vi "ArmPressureCalcMethod.vi"() -> ()   [LabVIEW 2013]
uses:
  Controls/Enum Save Action Events.ctl
  main.lvlib
panel:
  in  "SaveBtn":bool
  out "Description":string="Beregner det gennemsnitlige tryk ud fra alle de indtastede værdier for hver kolonne. "
  in  "Calculation Type":T1(ring) caption="Vælg metode til udregning af amtryk"
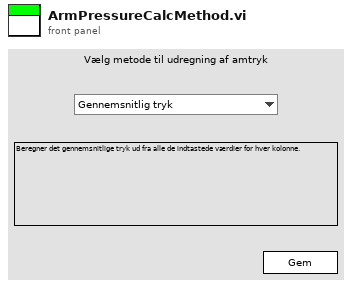
[diagram p1: front panel]
types:
  T1 = enum16{"Gennemsnitlig tryk", "Maksimalt tryk", "Dynamisk middel"}
  T2 = typedef "main.lvlib/Enum Save Action Events.ctl" = enum16{"LoadReportPath", "SaveReportPath", "Load Graph Path", "Save Graph Path", "LoadDataPath", "SaveDataPath", "Load Template Path", "Save Template Path", "Load PressureFactor", "Save PressureFactor", "Init", "Load Listbox", "Save Listbox", "LoadHospInfo", "SaveHospInfo", "Load DICOM Activation", "Save DICOM Activation", "LoadDICOMInfoWL", "SaveDICOMInfoWL", "LoadDICOMInfoPACS", "SaveDICOMInfoPACS", "Load ArmCalcMethod", "Save ArmCalcMethod", "LoadItemTags", "SaveItemTags", "LoadDICOMEncoding", "SaveDICOMEncoding", "LoadJournalType", "SaveJournalType", "LoadAcqFilterType", "SaveAcqFilterType", "Load Sequence", "Save Sequence", "Load Acquisition Mode", "Save Acquisition Mode", "Load General Settings", "Save General Settings", "Load Language", "Save Language", "Load Dicom Tags", "Save Dicom Tags", "Load BT Serial", "Save BT Serial", "Load BT License", "Save BT License"}
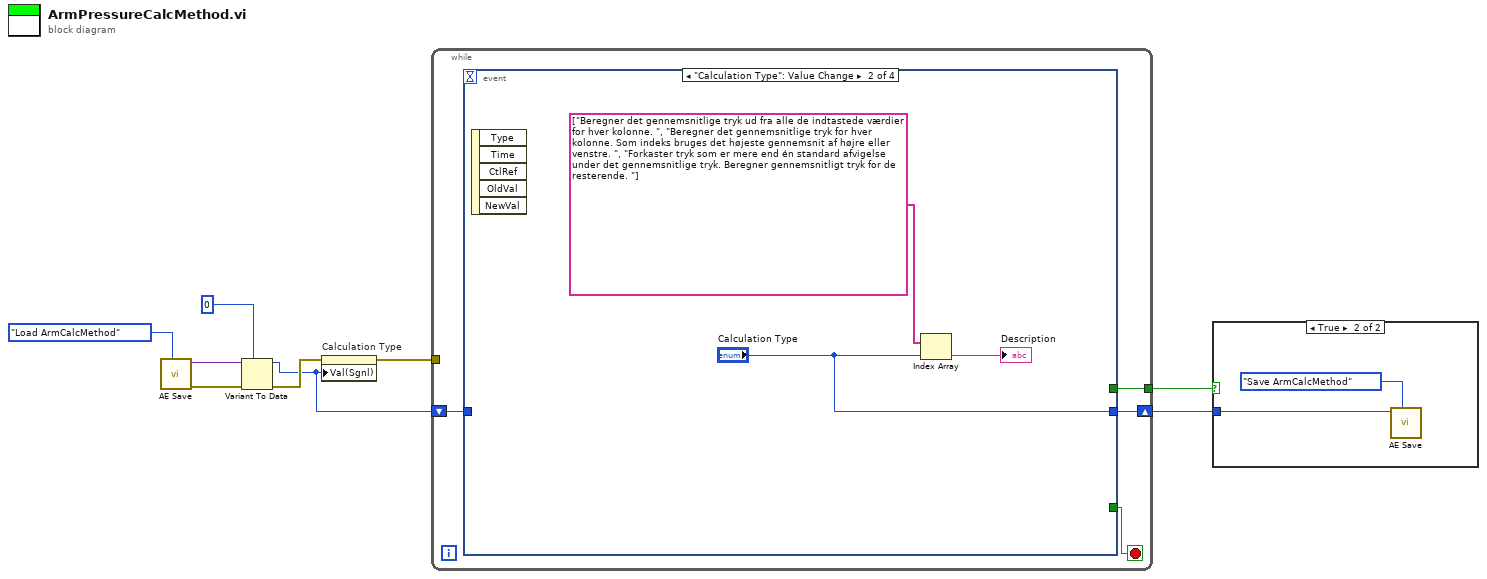
[diagram p0: block diagram]
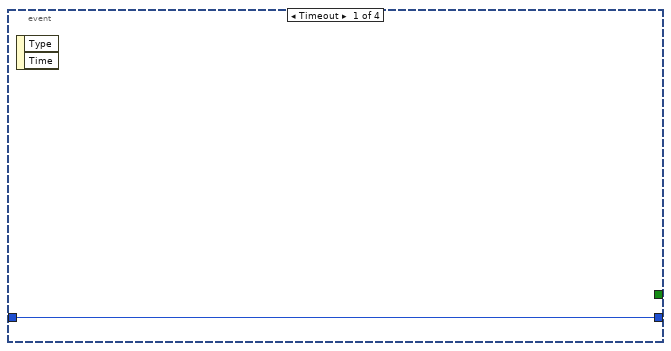
[diagram p3: hidden frame]
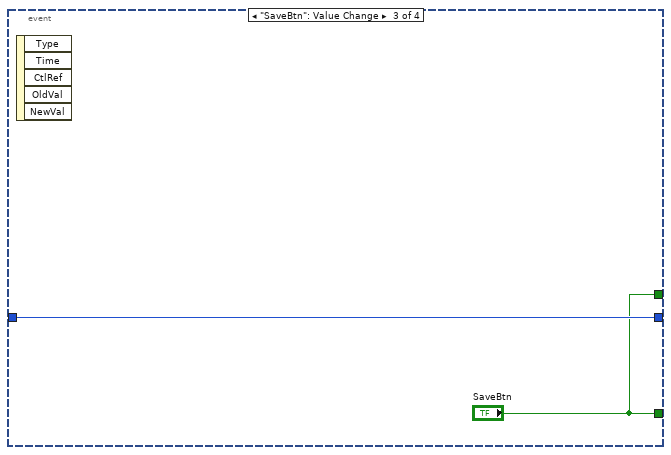
[diagram p4: hidden frame]
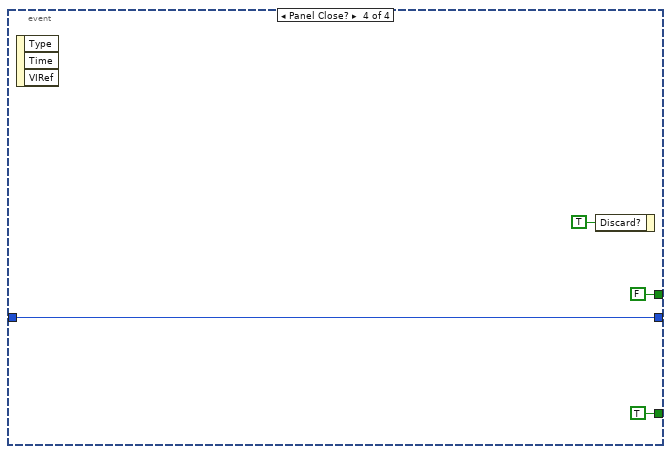
[diagram p5: hidden frame]
diagram:
  n1 = call "AE Save.vi"("Action"=Enum_Save_Action_Events."Load ArmCalcMethod") -> ("error out"=w5:errorcluster, "Anything"=w7:variant)  [unwired: 8 in]
  n2 = Variant To Data(error in=w5, type=0, Variant=w7) -> (data=w2:i32, error out=w4:errorcluster)
  n3 = property on="Calculation Type" class="Enum (strict)"(error in=w4, "Val(Sgnl)"=w2) -> (error out=w3:errorcluster)  [unwired: 1 in, 1 out]
  n4 = while {
    shift-right: [w12] -> w9
    shift-left: w2 -> [w11]
    tunnel: w3 -> [_]
    tunnel: [w10] -> w1
    stop <- w13 stop-if-true
    n5 = event shown="[1] \"Calculation Type\": Value Change" {
      selector: _ -> [_ _ _ _]
      dyn-events: _ -> [_ _ _ _]
      timeout: _ -> [_ _ _ _]
      tunnel: [_ _ "SaveBtn" TRUE ("SaveBtn")] -> w13
      tunnel: [w14 "Calculation Type" w19 w21] -> w12
      tunnel: w11 -> [w14 _ w19 w21]
      tunnel: [_ _ "SaveBtn" FALSE ("SaveBtn")] -> w10
      event Timeout {
        n6 = event-data() -> ()  [unwired: 1 in, 2 out]
      }
      event "Calculation Type": Value Change {
        n7 = event-data() -> ()  [unwired: 1 in, 5 out]
        n8 = Index Array(array=string[] ["Beregner det gennemsnitlige tryk ud fra alle de indtastede værdier for hver kolonne. ", "Beregner det gennemsnitlige tryk for hver kolonne. Som indeks bruges det højeste gennemsnit af højre eller venstre. ", "Forkaster tryk som er mere end én standard afvigelse under det gennemsnitlige tryk. Beregner gennemsnitligt tryk for de resterende. "], index="Calculation Type") -> (element=→"Description":string)
      }
      event "SaveBtn": Value Change {
        n9 = event-data() -> ()  [unwired: 1 in, 5 out]
      }
      event Panel Close? {
        n10 = event-data() -> ()  [unwired: 1 in, 3 out]
        n11 = event-data("Discard?"=TRUE) -> ()  [unwired: 1 in, 1 out]
      }
    }
  }
  n12 = case shown="True" w1 {
    tunnel: w9 -> [_ w24]
    frame False {
    }
    frame True {
      n13 = call "AE Save.vi"("Variant In"=w24, "Action"=Enum_Save_Action_Events."Save ArmCalcMethod") -> ()  [unwired: 7 in, 2 out]
    }
  }
